vi "LinearControl.vi"(6 "Loop Iteration":i32, 8 "Reset":bool, 9 "Rate (unit/s)":dbl=0.5, 10 "Setpoint":dbl, 11 "Motor Value":dbl) -> (0 "Currently Matching":bool, 3 "New Motor Value":dbl)   [LabVIEW 2012]
doc: "Changes a given motor value based on time since last call, given rate, and given set point. Rate of change is always linear with respect to time. Designed to be run multiple times in while loop. Use shift register to maintain Motor Value in external while loop."
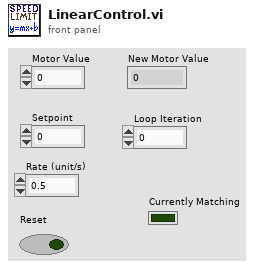
[diagram p1: front panel]
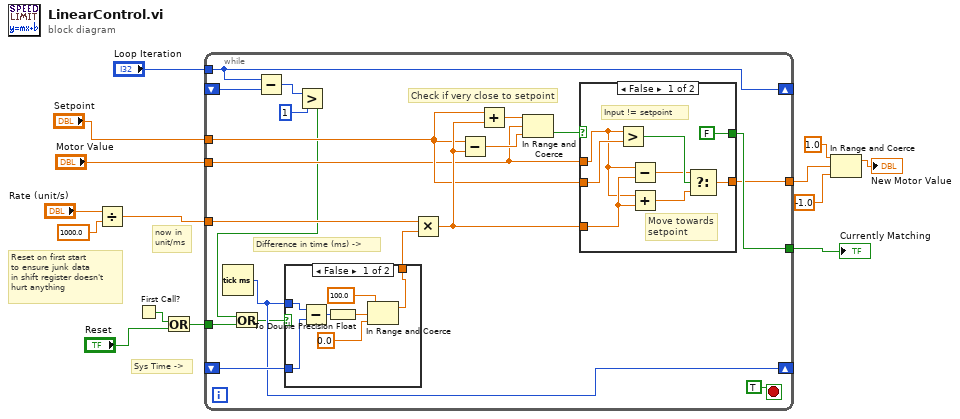
[diagram p0: block diagram]
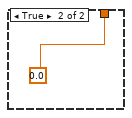
[diagram p2: hidden frame]
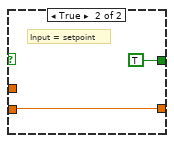
[diagram p3: hidden frame]
diagram:
  # "Reset on first start\nto ensure junk data\nin shift register doesn't\nhurt anything"
  # "now in\nunit/ms"
  # "Sys Time ->"
  n1 = Divide(x="Rate (unit/s)", y=1000.0) -> (x/y=w11:dbl)
  n2 = First Call?() -> (First Call?: T/F=w9:bool)
  n3 = Or(x=w9, y="Reset") -> (x .or. y?=w7:bool)
  n4 = while {
    tunnel: w11 -> [w32]
    tunnel: [w34] -> w14
    tunnel: "Setpoint" -> [w30]
    tunnel: w7 -> [w17]
    shift-right: [w26] -> _
    shift-left: _ -> [w27]
    tunnel: "Motor Value" -> [w23]
    tunnel: [w22] -> w5
    shift-right: [w18] -> _
    shift-left: _ -> [w21]
    tunnel: "Loop Iteration" -> [w18]
    stop <- TRUE stop-if-true
    # "Difference in time (ms) ->"
    # "Check if very close to setpoint"
    n5 = Tick Count (ms)() -> (millisecond timer value=w26:u32)
    n6 = Subtract(x=w18, y=w21) -> (x-y=w20:i32)
    n7 = Greater?(x=w20, y=1) -> (0:w15:bool)
    n8 = Or(x=w15, y=w17) -> (x .or. y?=w16:bool)
    n9 = case shown="False" w16 {
      tunnel: w27 -> [w40 _]
      tunnel: w26 -> [w41 _]
      tunnel: [w35 0.0] -> w25
      frame False {
        n10 = Subtract(x=w41, y=w40) -> (x-y=w39:u32)
        n11 = To Double Precision Float(number=w39) -> (double precision float=w38:dbl)
        n12 = In Range and Coerce(upper limit=100.0, x=w38, lower limit=0.0) -> (coerced(x)=w35:dbl)  [unwired: 1 out]
      }
      frame True {
      }
    }
    n13 = Multiply(x=w32, y=w25) -> (x*y=w31:dbl)
    n14 = Subtract(x=w30, y=w31) -> (x-y=w24:dbl)
    n15 = Add(x=w30, y=w31) -> (x+y=w29:dbl)
    n16 = In Range and Coerce(upper limit=w29, x=w23, lower limit=w24) -> (In Range?=w28:bool)  [unwired: 1 out]
    n17 = case shown="False" w28 {
      tunnel: [w45 w51] -> w22
      tunnel: w31 -> [w47 _]
      tunnel: [FALSE TRUE] -> w34
      tunnel: w30 -> [w44 w51]
      tunnel: w23 -> [w43 _]
      frame False {
        # "Move towards\nsetpoint"
        # "Input != setpoint"
        n18 = Greater?(x=w43, y=w44) -> (0:w49:bool)
        n19 = Subtract(x=w43, y=w47) -> (x-y=w48:dbl)
        n20 = Add(x=w43, y=w47) -> (x+y=w46:dbl)
        n21 = Select(t=w48, s=w49, f=w46) -> (s? t:f=w45:dbl)
      }
      frame True {
        # "Input = setpoint"
      }
    }
  }
  "Currently Matching" <- w14
  n22 = In Range and Coerce(upper limit=1.0, x=w5, lower limit=-1.0) -> (coerced(x)=→"New Motor Value":dbl)  [unwired: 1 out]
